vi "Initialize_Graph.vi"(11 "XYGraph in":refnum<vi>) -> (0 "error out":errorcluster)   [LabVIEW 2017]
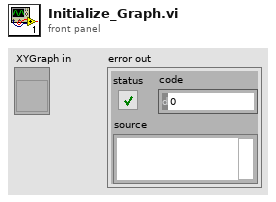
[diagram p1: front panel]
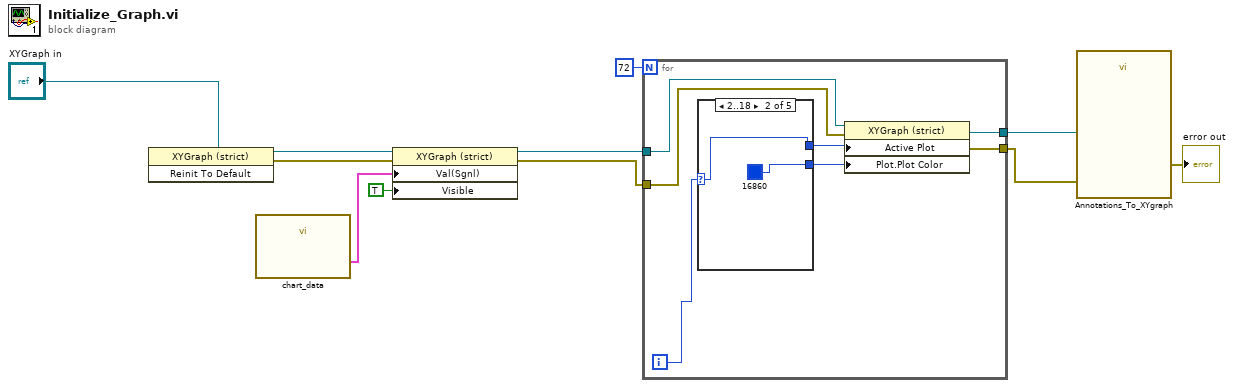
[diagram p0: block diagram]
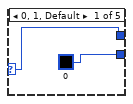
[diagram p2: hidden frame]
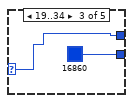
[diagram p3: hidden frame]
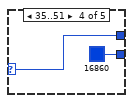
[diagram p4: hidden frame]
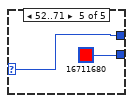
[diagram p5: hidden frame]
diagram:
  n1 = invoke class="XYGraph (strict)" method="Reinit To Default"(reference="XYGraph in") -> (reference out=w8:refnum<vi>, error out=w9:errorcluster)  [unwired: 2 in, 1 out]
  n2 = call "chart_data.vi"() -> ("Output Graphs"=w11:cluster{"all rows":dbl[], "all rows":dbl[]}[])  [unwired: 9 in]
  n3 = property class="XYGraph (strict)"(reference=w8, error in=w9, "Val(Sgnl)"=w11, "Visible"=TRUE) -> (reference out=w6:refnum<vi>, error out=w5:errorcluster)
  n4 = for {
    N: 72 -> [_]
    tunnel: w6 -> [w15]
    tunnel: w5 -> [w14]
    tunnel: [w16] -> w3
    tunnel: [w17] -> w2
    i -> [w18]
    n5 = case shown="2..18" w18 {
      selector: w18 -> [w19 w21 w23 w25 w27]
      tunnel: [u32 0 u32 16860 u32 16860 u32 16860 u32 16711680] -> w13
      tunnel: [w19 w21 w23 w25 w27] -> w12
      frame 0, 1, Default {
      }
      frame 2..18 {
      }
      frame 19..34 {
      }
      frame 35..51 {
      }
      frame 52..71 {
      }
    }
    n6 = property class="XYGraph (strict)"(reference=w15, error in=w14, "Active Plot"=w12, "Plot.Plot Color"=w13) -> (reference out=w17:refnum<vi>, error out=w16:errorcluster)
  }
  n7 = call "Annotations_To_XYgraph.vi"("error in (no error)"=w3, "XYGraph in"=w2) -> ("error out"=→"error out":errorcluster)  [unwired: 8 in, 1 out]
